vi "SWERVE_MODULE_ACT.vi"(9 "Swerve Sense":T2={"Speed"=0.0, "Angle"={"VALUE"=0.0, "COS"=1.0, "SIN"=0.0}} {"Angle"."SIN" format="%13.4f"; "Angle"."COS" format="%13.4f"; "Angle"."VALUE" format="%13.4f"}, 10 "Swerve Dmd":T2={"Speed"=0.0, "Angle"={"VALUE"=0.0, "COS"=1.0, "SIN"=0.0}} {"Angle"."SIN" format="%13.4f"; "Angle"."COS" format="%13.4f"; "Angle"."VALUE" format="%13.4f"}, 11 "Swerve Module TypDef":T4) -> (2 "Swerve Motor Dmd":dbl, 3 "Wheel Motor Dmd":dbl)   [LabVIEW 2019]
uses:
  SWERVE_MODULE_TYPDEF.ctl
  <vilib>/Rock Robotics/WPI/MotorControl/WPI_MotorControlDeviceRef.ctl
  <vilib>/Rock Robotics/WPI/MotorControl/WPI_MotorControlType.ctl
  <vilib>/Rock Robotics/SystemInterfaces/DIO/FPGA_DIOPWMChannel.ctl
  <vilib>/Rock Robotics/WPI/PWM/WPI_PWMDeadband.ctl
  <vilib>/Rock Robotics/SystemInterfaces/DIO/FPGA_DIOChannel.ctl
  <vilib>/Rock Robotics/WPI/Encoder/WPI_EncoderDevRef.ctl
  <vilib>/Rock Robotics/SystemInterfaces/Encoder/FPGA_EncoderIdx.ctl
  <vilib>/Rock Robotics/SystemInterfaces/Counter/FPGA_CounterCtrSystemIndex.ctl
  <vilib>/Rock Robotics/WPI/Encoder/WPI_EncoderType.ctl
  <vilib>/Rock Robotics/WPI/ThirdParty/JAS_Junk/TrajLib/SWERVE_DRIVE_MODULE_STATE.ctl
  <vilib>/Rock Robotics/WPI/ThirdParty/JAS_Junk/TrajLib/ROTATION2D.ctl
  SWERVE_MODULE_MOTOR_CO.ctl
  <vilib>/addons/control/pid/pid.llb/PID (DBL).vi
  <vilib>/addons/control/pid/NI_PID_pid.lvlib
  Secret_Control_Library_Protected/Secret_Control_Library_Protected.lvlib
  <vilib>/Rock Robotics/WPI/ThirdParty/JAS_Junk/TrajLib/Trajectory_Library.lvlib
panel:
  in  "Speed PID":T1={"proportional gain (Kc)"=0.45, "integral time (Ti, min)"=0.008, "derivative time (Td, min)"=0.0} {"derivative time (Td, min)" format="%.3f"; "integral time (Ti, min)" format="%.3f"; "proportional gain (Kc)" format="%.3f"}
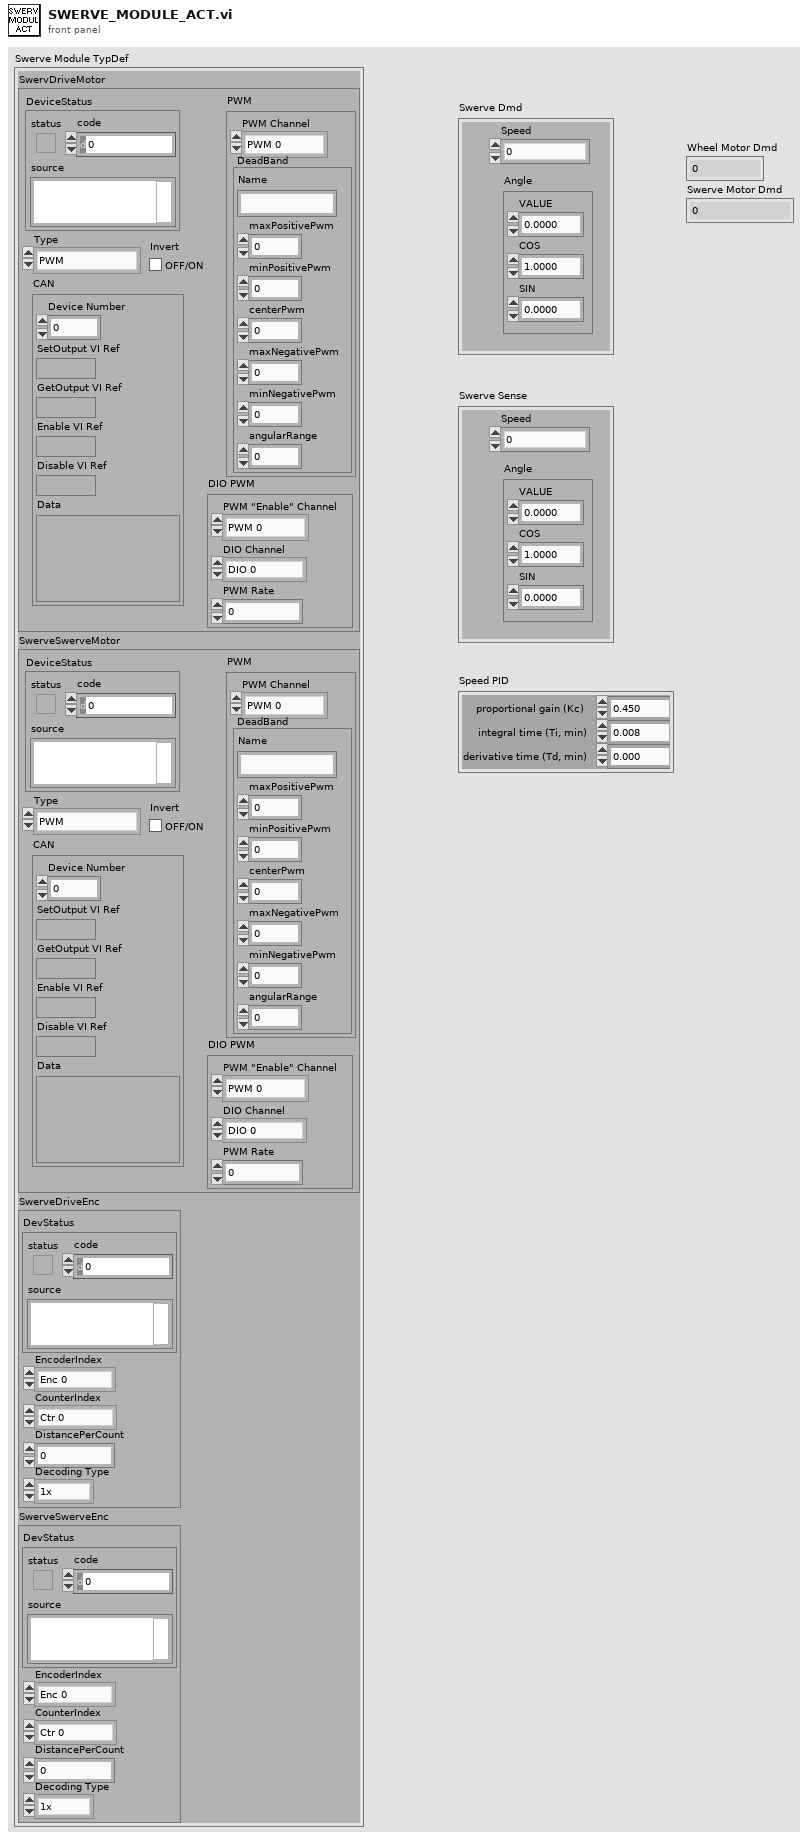
[diagram p1: front panel]
types:
  T1 = cluster{"proportional gain (Kc)":dbl, "integral time (Ti, min)":dbl, "derivative time (Td, min)":dbl}
  T2 = typedef "Trajectory_Library.lvlib/SWERVE_DRIVE_MODULE_STATE.ctl" = cluster{"Speed":dbl, "Angle":T3}
  T3 = typedef "Trajectory_Library.lvlib/ROTATION2D.ctl" = cluster{"VALUE":dbl, "COS":dbl, "SIN":dbl}
  T4 = typedef "SWERVE_MODULE_TYPDEF.ctl" = cluster{"SwervDriveMotor":T5, "SwerveSwerveMotor":T5, "SwerveDriveEnc":T10, "SwerveSwerveEnc":T10}
  T5 = typedef "WPI_MotorControlDeviceRef.ctl" = cluster{"DeviceStatus":errorcluster, "Type":T6, "PWM":cluster{"PWM Channel":T7, "DeadBand":T8}, "CAN":cluster{"Device Number":u8, "SetOutput VI Ref":variant, "GetOutput VI Ref":variant, "Enable VI Ref":variant, "Disable VI Ref":variant, "Data":variant}, "Invert":bool, "DIO PWM":cluster{"PWM \"Enable\" Channel":T7, "DIOChannel":T9, "PWM Rate":dbl}}
  T6 = typedef "WPI_MotorControlType.ctl" = enum16{"PWM", "CAN", "DIO PWM"}
  T7 = typedef "FPGA_DIOPWMChannel.ctl" = enum8{"PWM 0", "PWM 1", "PWM 2", "PWM 3", "PWM 4", "PWM 5", "PWM 6", "PWM 7", "PWM 8", "PWM 9", "PWM MXP 0", "PWM MXP 1", "PWM MXP 2", "PWM MXP 3", "PWM MXP 4", "PWM MXP 5", "PWM MXP 6", "PWM MXP 7", "PWM MXP 8", "PWM MXP 9", "Invalid"}
  T8 = typedef "WPI_PWMDeadband.ctl" = cluster{"Name":string, "maxPositivePwm":i32, "minPositivePwm":i32, "centerPwm":i32, "maxNegativePwm":i32, "minNegativePwm":i32, "angularRange":u16}
  T9 = typedef "FPGA_DIOChannel.ctl" = enum8{"DIO 0", "DIO 1", "DIO 2", "DIO 3", "DIO 4", "DIO 5", "DIO 6", "DIO 7", "DIO 8", "DIO 9", "DIO MXP 0", "DIO MXP 1", "DIO MXP 2", "DIO MXP 3", "DIO MXP 4", "DIO MXP 5", "DIO MXP 6", "DIO MXP 7", "DIO MXP 8", "DIO MXP 9", "DIO MXP 10", "DIO MXP 11", "DIO MXP 12", "DIO MXP 13", "DIO MXP 14", "DIO MXP 15", "SPI Port CS1", "SPI Port CS2", "SPI Port CS3", "SPI Port MISO", "SPI Port MOSI", "Invalid"}
  T10 = typedef "WPI_EncoderDevRef.ctl" = cluster{"DevStatus":errorcluster, "EncoderIndex":T11, "CounterIndex":T12, "DistancePerCount":dbl, "Decoding Type":T13}
  T11 = typedef "FPGA_EncoderIdx.ctl" = enum8{"Enc 0", "Enc 1", "Enc 2", "Enc 3", "Enc 4", "Enc 5", "Enc 6", "Enc 7", "Invalid"}
  T12 = typedef "FPGA_CounterCtrSystemIndex.ctl" = enum8{"Ctr 0", "Ctr 1", "Ctr 2", "Ctr 3", "Ctr 4", "Ctr 5", "Ctr 6", "Ctr 7", "Invalid"}
  T13 = typedef "WPI_EncoderType.ctl" = enum16{"1x", "2x", "4x"}
  T14 = typedef "SWERVE_MODULE_MOTOR_CO.ctl" = cluster{"WheelMotorDmd":dbl, "SwerveMotorDmd":dbl}
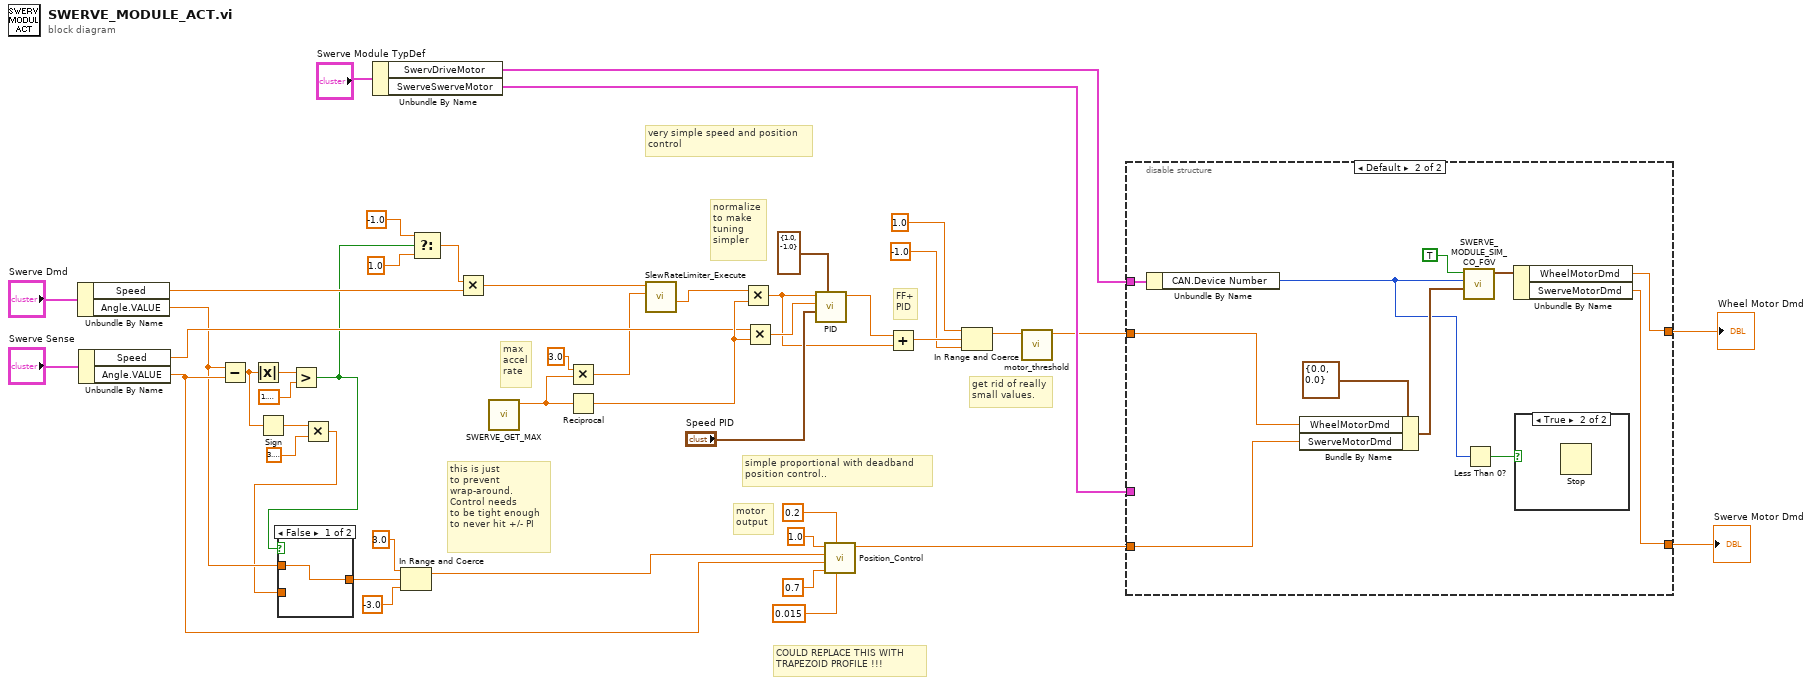
[diagram p0: block diagram]
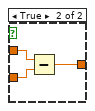
[diagram p2: hidden frame]
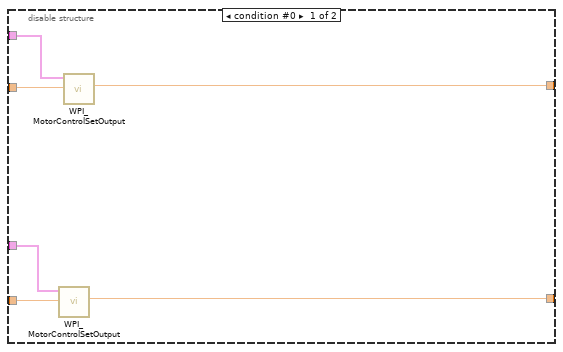
[diagram p3: hidden frame]
diagram:
  # "COULD REPLACE THIS WITH\nTRAPEZOID PROFILE !!!"
  # "simple proportional with deadband\nposition control.."
  # "motor\noutput"
  # "this is just\nto prevent\nwrap-around.\nControl needs\nto be tight enough\nto never hit +/- PI"
  # "very simple speed and position\ncontrol"
  # "get rid of really\nsmall values."
  # "max\naccel\nrate"
  # "normalize\nto make\ntuning\nsimpler"
  # "FF+\nPID"
  n1 = Unbundle By Name("Swerve Dmd") -> ("Speed"=w13:dbl, "Angle.VALUE"=w7:dbl)
  n2 = Unbundle By Name("Swerve Sense") -> ("Speed"=w31:dbl, "Angle.VALUE"=w17:dbl)
  n3 = Subtract(x=w7, y=w17) -> (x-y=w10:dbl)
  n4 = Absolute Value(x=w10) -> (abs(x)=w16:dbl)
  n5 = Sign(1:w10) -> (0:w9:dbl)
  n6 = Greater?(x=w16, y=1.5707963267948966) -> (0:w4:bool)
  n7 = Multiply(x=w9, y=3.141592653589793) -> (x*y=w6:dbl)
  n8 = case shown="False" w4 {
    tunnel: w7 -> [w47 w50]
    tunnel: w6 -> [_ w49]
    tunnel: [w47 w48] -> w5
    frame False {
    }
    frame True {
      n9 = Subtract(x=w50, y=w49) -> (x-y=w48:dbl)
    }
  }
  n10 = Unbundle By Name("Swerve Module TypDef") -> ("SwervDriveMotor"=w20:T5, "SwerveSwerveMotor"=w22:T5)
  n11 = In Range and Coerce(upper limit=3.0, x=w5, lower limit=-3.0) -> (coerced(x)=w28:dbl)  [unwired: 1 out]
  n12 = Select(t=-1.0, s=w4, f=1.0) -> (s? t:f=w12:dbl)
  n13 = Multiply(x=w12, y=w13) -> (x*y=w2:dbl)
  n14 = call "SWERVE_GET_MAX.vi"() -> ("Max Wheel Vel (Meter/Sec)"=w34:dbl)  [unwired: 10 in, 1 out]
  n15 = Multiply(x=3.0, y=w34) -> (x*y=w1:dbl)
  n16 = Reciprocal(x=w34) -> (1/x=w36:dbl)
  n17 = call <vilib>:"SlewRateLimiter_Execute.vi"("Rate"=w1, "Input"=w2) -> ("Output"=w3:dbl)  [unwired: 8 in, 1 out]
  n18 = Multiply(x=w3, y=w36) -> (x*y=w38:dbl)
  n19 = Multiply(x=w31, y=w36) -> (x*y=w39:dbl)
  n20 = call-poly <vilib>:"PID.vi"("output range"=cluster{"output high":dbl, "output low":dbl} {"output high"=1.0, "output low"=-1.0}, "PID gains"="Speed PID", "process variable"=w39, "setpoint"=w38) -> ("output"=w45:dbl)  [unwired: 6 in, 1 out]
  n21 = call "Position_Control.vi"("ErrDeadband"=0.015, "MinOutput"=0.2, "ErrThreshold"=0.7, "CurrentPosition"=w17, "TargetPosition"=w28, "MaxOutput"=1.0) -> ("Output"=w23:dbl)  [unwired: 3 in, 2 out]
  n22 = Add(x=w45, y=w38) -> (x+y=w44:dbl)
  n23 = In Range and Coerce(upper limit=1.0, x=w44, lower limit=-1.0) -> (coerced(x)=w35:dbl)  [unwired: 1 out]
  n24 = call "motor_threshold.vi"("motor in"=w35) -> ("motor out"=w21:dbl)  [unwired: 10 in]
  n25 = disable-structure shown="Default" {
    disable-tunnel: w23 -> [w56 w63]
    disable-tunnel: w22 -> [w55 _]
    disable-tunnel: w21 -> [w54 w64]
    disable-tunnel: w20 -> [w53 w67]
    disable-tunnel: [w52 w58] -> w19
    disable-tunnel: [w51 w57] -> w18
    frame condition #0 {
      n26 = call <vilib>:"WPI_MotorControlSetOutput.vi"("Output"=w56, "MotorControlDevRef"=w55) -> ("Motor Output"=w51:dbl)  [unwired: 7 in, 2 out]
      n27 = call <vilib>:"WPI_MotorControlSetOutput.vi"("Output"=w54, "MotorControlDevRef"=w53) -> ("Motor Output"=w52:dbl)  [unwired: 7 in, 2 out]
    }
    frame condition #1 (active) {
      n28 = Unbundle By Name(w67) -> ("CAN.Device Number"=w60:u8)
      n29 = Bundle By Name(cluster=T14 {"WheelMotorDmd"=0.0, "SwerveMotorDmd"=0.0} ("SwerveModuleMotorDmd"), "WheelMotorDmd"=w64, "SwerveMotorDmd"=w63) -> (w62:T14)
      n30 = call "SWERVE_MODULE_SIM_CO_FGV.vi"("in SwerveModuleMotorDmd"=w62, "Index"=w60, "WRITE"=TRUE) -> ("out SwerveModuleMotorDmd"=w59:T14)  [unwired: 8 in]
      n31 = Less Than 0?(x=w60) -> (x < 0?=w61:bool)
      n32 = Unbundle By Name(w59) -> ("WheelMotorDmd"=w58:dbl, "SwerveMotorDmd"=w57:dbl)
      n33 = case shown="True" w61 {
        frame False {
        }
        frame True {
          n34 = Stop() -> ()  [unwired: 1 in]
        }
      }
    }
  }
  "Wheel Motor Dmd" <- w19
  "Swerve Motor Dmd" <- w18
